vi "Loop_HW Line.vi"() -> ()   [LabVIEW 2017, in "Hopper System.lvlib"]
uses:
  Hopper System.lvlib
  <vilib>/Rock Robotics/SystemInterfaces/DIO/FPGA_DIOChannel.ctl
  Globals/Global_STOP.vi
  Global_HW Status.vi
  Globals/Global_Hopper Statis.vi
panel:
  out "Ball Shot":bool
  out "Ball Present":bool
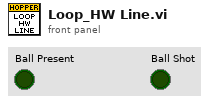
[diagram p1: front panel]
types:
  T1 = typedef "FPGA_DIOChannel.ctl" = enum8{"DIO 0", "DIO 1", "DIO 2", "DIO 3", "DIO 4", "DIO 5", "DIO 6", "DIO 7", "DIO 8", "DIO 9", "DIO MXP 0", "DIO MXP 1", "DIO MXP 2", "DIO MXP 3", "DIO MXP 4", "DIO MXP 5", "DIO MXP 6", "DIO MXP 7", "DIO MXP 8", "DIO MXP 9", "DIO MXP 10", "DIO MXP 11", "DIO MXP 12", "DIO MXP 13", "DIO MXP 14", "DIO MXP 15", "SPI Port CS1", "SPI Port CS2", "SPI Port CS3", "SPI Port MISO", "SPI Port MOSI", "Invalid"}
  T2 = typedef "WPI_DigitalInputDevRef.ctl" = cluster{"DevStatus":errorcluster, "DIO Channel":T1}
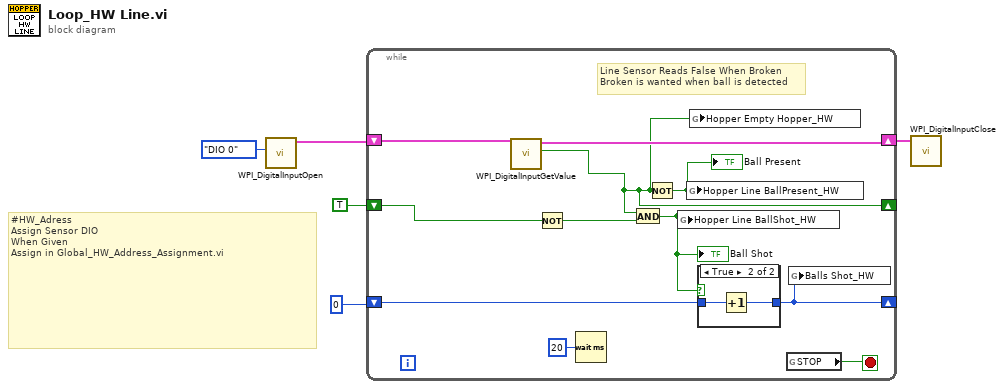
[diagram p0: block diagram]
diagram:
  # "#HW_Adress\nAssign Sensor DIO\nWhen Given\nAssign in Global_HW_Address_Assignment.vi"
  n1 = call <vilib>:"WPI_DigitalInputOpen.vi"("DIO Channel"=FPGA_DIOChannel."DIO 0") -> ("DigitalInputDevRef"=w5:T2)  [unwired: 9 in, 1 out]
  n2 = while {
    shift-right: [w15] -> w4
    shift-left: w5 -> [w10]
    shift-right: [w6] -> _
    shift-left: TRUE -> [w12]
    shift-right: [w7] -> _
    shift-left: 0 -> [w8]
    stop <- w16 stop-if-true
    # "Line Sensor Reads False When Broken\nBroken is wanted when ball is detected"
    n3 = call <vilib>:"WPI_DigitalInputGetValue.vi"("DigitalInputDevRef"=w10) -> ("Value"=w6:bool, "DigitalInputDevRef"=w15:T2)  [unwired: 8 in, 1 out]
    n4 = Not(x=w12) -> (.not. x?=w13:bool)
    n5 = Wait (ms)(milliseconds to wait=u32 20) -> ()  [unwired: 1 out]
    n6 = And(x=w6, y=w13) -> (x .and. y?=w9:bool)
    "Ball Shot" <- w9
    n7 = Not(x=w6) -> (.not. x?=w11:bool)
    "Ball Present" <- w11
    n8 = global write "Global_HW Status.vi" "Hopper Line BallShot_HW"(w9) -> ()
    n9 = global write "Global_HW Status.vi" "Hopper Line BallPresent_HW"(w11) -> ()
    n10 = global write "Global_Hopper Statis.vi" "Hopper Empty Hopper_HW"(w6) -> ()
    n11 = case shown="True" w9 {
      tunnel: w8 -> [w17 w19]
      tunnel: [w17 w18] -> w7
      frame False {
      }
      frame True {
        n12 = Increment(x=w19) -> (x+1=w18:i32)
      }
    }
    n13 = global read "Global_STOP.vi" "STOP"() -> (w16:bool)
    n14 = global write "Global_HW Status.vi" "Balls Shot_HW"(w7) -> ()
  }
  n15 = call <vilib>:"WPI_DigitalInputClose.vi"("DigitalInputDevRef"=w4) -> ()  [unwired: 10 in, 1 out]
